vi "Go At Angle.vi"(0 "Target Angle":dbl=1.9971579416928176, 1 "Speed":T2={"\nMoving speed"=0.3728813559322034, "Turning speed limit"=1.0296610169491527} {"Turning speed limit" scale=0.0..4.5; "Moving speed" scale=0.0..4.5}, 2 "Bot Angle":dbl=2.422342777629885, 3 "dt":dbl=0.03, 5 "Stop motors":bool=TRUE) -> ()   [LabVIEW 2017]
uses:
  <vilib>/addons/control/pid/pid.llb/PID (DBL).vi
  <vilib>/addons/control/pid/NI_PID_pid.lvlib
panel:
  in  "PID gains":T1={"proportional gain (Kc)"=0.6, "integral time (Ti, min)"=0.0, "derivative time (Td, min)"=0.001} {"derivative time (Td, min)" format="%.7f"; "integral time (Ti, min)" format="%.7f"; "proportional gain (Kc)" format="%.7f"}
  in  "threshold angle":dbl=0.15
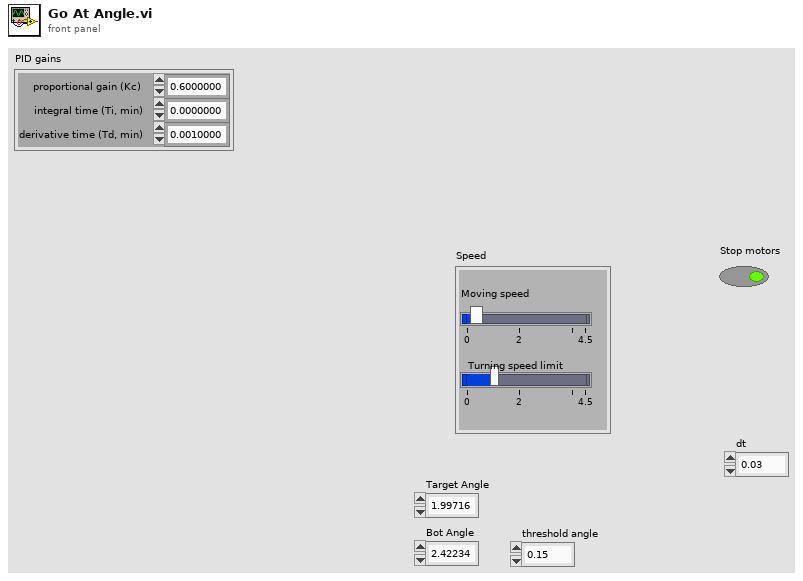
[diagram p1: front panel]
types:
  T1 = cluster{"proportional gain (Kc)":dbl, "integral time (Ti, min)":dbl, "derivative time (Td, min)":dbl}
  T2 = cluster{"\nMoving speed":dbl, "Turning speed limit":dbl}
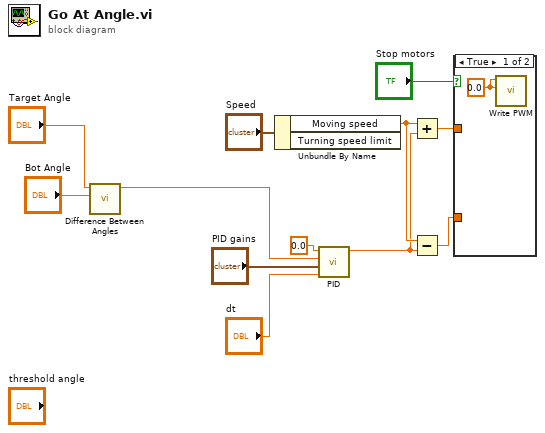
[diagram p0: block diagram]
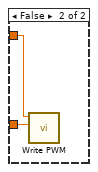
[diagram p2: hidden frame]
diagram:
  n1 = call "Difference Between Angles.vi"("Angle 2"="Bot Angle", "Angle 1"="Target Angle") -> ("Difference"=w7:dbl)  [unwired: 9 in]
  n2 = Unbundle By Name("Speed") -> ("Moving speed"=w4:dbl)  [unwired: 1 out]
  n3 = call-poly <vilib>:"PID.vi"("dt (s)"="dt", "PID gains"="PID gains", "process variable"=w7, "setpoint"=0.0) -> ("output"=w3:dbl)  [unwired: 6 in, 1 out]
  n4 = Add(x=w4, y=w3) -> (x+y=w2:dbl)
  n5 = Subtract(x=w4, y=w3) -> (x-y=w1:dbl)
  n6 = case shown="True" "Stop motors" {
    tunnel: w2 -> [_ w15]
    tunnel: w1 -> [_ w14]
    frame True {
      w13 = 0.0 ("Left")
      n7 = call "Write PWM.vi"("Left"=w13, "Right"=w13) -> ()  [unwired: 8 in]
    }
    frame False {
      n8 = call "Write PWM.vi"("Left"=w15, "Right"=w14) -> ()  [unwired: 8 in]
    }
  }
